vi "HGF_SVVisitor_register.appendData2Variant.vi"(0 "variant":variant, 1 "Shared Variable Control (DSC)":refnum<k21>, 2 "HGF_NetworkVisitor":refnum<class "HGF_NetworkVisitor.lvclass">, 3 "HGF_TriggeredEvent":refnum<class "HGF_TriggeredEvent.lvclass">, 4 "shared variable refnum (without DSC)":refnum<k21>, 5 "error in":errorcluster) -> (14 "dup variant":variant, 19 "error out":errorcluster)   [LabVIEW 2012, in "HGF_SV.lvlib" / "HGF_SVMonitorVisitor_register.lvclass"]
uses:
  HGF_SVMonitorVisitor_register.lvclass
  HGF_BaseClasses/HGF_NetworkVisitor/HGF_NetworkVisitor.lvclass
  HGF_BaseClasses/HGF_TriggeredEvent/HGF_TriggeredEvent.lvclass
  <resource>/objmgr/ni.var.rc
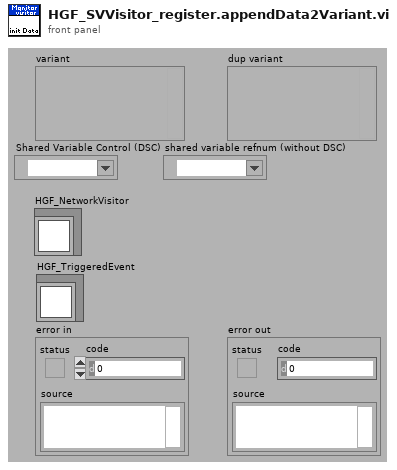
[diagram p1: front panel]
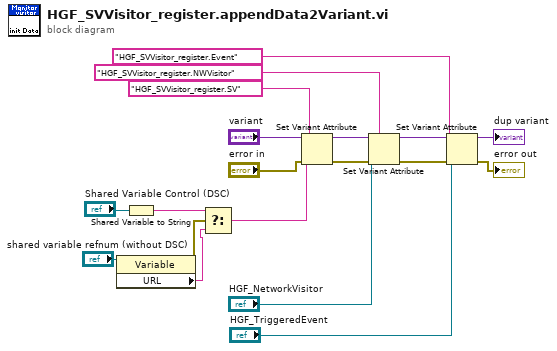
[diagram p0: block diagram]
diagram:
  n1 = property class="Variable"(reference="shared variable refnum (without DSC)") -> (error out=w1:errorcluster, "URL"=w5:string)  [unwired: 1 in, 1 out]
  n2 = Shared Variable to String(1:"Shared Variable Control (DSC)") -> (0:w6:string)
  n3 = Select(t=w6, s=w1, f=w5) -> (s? t:f=w4:string)
  n4 = Set Variant Attribute(Variant="variant", name="HGF_SVVisitor_register.SV", value=w4, error in="error in") -> (Variant out=w17:variant, error out=w11:errorcluster)  [unwired: 1 out]
  n5 = Set Variant Attribute(Variant=w17, name="HGF_SVVisitor_register.NWVisitor", value="HGF_NetworkVisitor", error in=w11) -> (Variant out=w16:variant, error out=w12:errorcluster)  [unwired: 1 out]
  n6 = Set Variant Attribute(Variant=w16, name="HGF_SVVisitor_register.Event", value="HGF_TriggeredEvent", error in=w12) -> (Variant out=→"dup variant":variant, error out=→"error out":errorcluster)  [unwired: 1 out]
